vi "Normalize Motor Velocity.vi"(11 "velocity (rad/s)":fxp<+/-,32,11>) -> (3 "normalized velocity":fxp<+/-,16,16>)   [LabVIEW 2011]
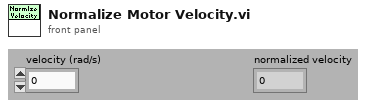
[diagram p1: front panel]
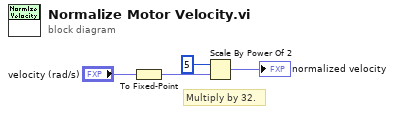
[diagram p0: block diagram]
diagram:
  # "Multiply by 32."
  n1 = To Fixed-Point(number="velocity (rad/s)") -> (fixed-point=w1:fxp<+/-,16,16>)  [unwired: 1 in]
  n2 = Scale By Power Of 2(n=5, x=w1) -> (x*2^n=→"normalized velocity":fxp<+/-,16,16>)
